vi "subVI QCam Change Image Type.vi"(2 "error in":errorcluster, 3 "Image In":T1, 4 "cameraId In":u32) -> (0 "error out":errorcluster, 1 "cameraId out":u32)   [LabVIEW 2012]
uses:
  <vilib>/vision/Image Controls.llb/IMAQ Image.ctl
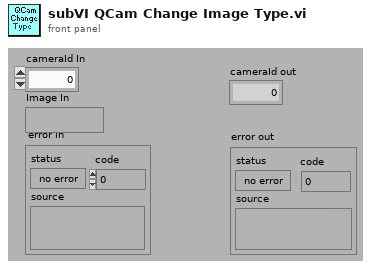
[diagram p1: front panel]
types:
  T1 = typedef "IMAQ Image.ctl" = refnum<image>
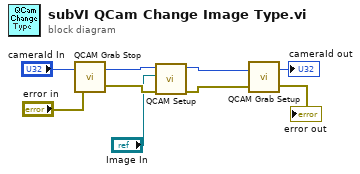
[diagram p0: block diagram]
diagram:
  n1 = call "QCAM Grab Stop.vi"("error in (no error)"="error in", "cameraId"="cameraId In") -> ("error out"=w2:errorcluster, "cameraId Out"=w3:u32)
  n2 = call <userlib>:"QCAM Setup.vi"("error in (no error)"=w2, "Image"="Image In", "cameraId"=w3) -> ("error out"=w4:errorcluster, "cameraId out"=w5:u32)  [unwired: 3 in, 4 out]
  n3 = call <userlib>:"QCAM Grab Setup.vi"("error in (no error)"=w4, "cameraId"=w5) -> ("error out"=→"error out":errorcluster, "cameraId out"=→"cameraId out":u32)
